vi "TTA_MATLAB_RFIC_Init.vi"(11 "error in":errorcluster) -> (4 "SuccessComm":bool[](array[boolean]), 15 "error out":errorcluster)   [LabVIEW 2016]
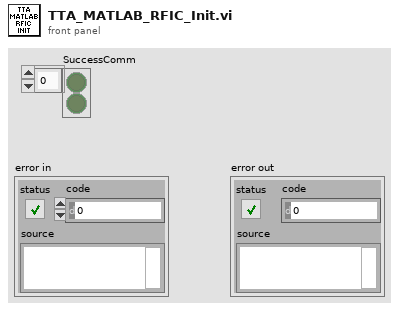
[diagram p1: front panel]
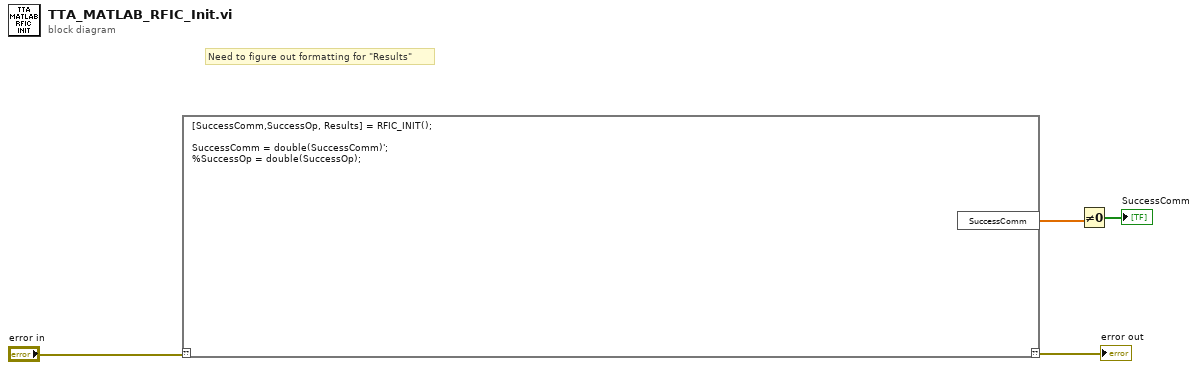
[diagram p0: block diagram]
diagram:
  # "Need to figure out formatting for \"Results\""
  n1 = script code="[SuccessComm,SuccessOp, Results] = RFIC_INIT();\n\nSuccessComm = double(SuccessComm)';\n%SuccessOp = double(SuccessOp);"("??"="error in") -> ("??"=→"error out":errorcluster, "SuccessComm"=w3:dbl[])
  n2 = Not Equal To 0?(x=w3) -> (x != 0?=→"SuccessComm":bool[])
